vi "LaudaDAQ.vi"(7 "device name":tag="cDAQ9188XT-1C3BF2FMod1") -> (0 "error out":errorcluster, 1 "Tj out":dbl, 2 "data":dynamicdata(waveform), 3 "Sensor OK":bool, 4 "Tj out":dbl, 5 "T external 2":dbl)   [LabVIEW 2016]
panel:
  out "Numeric":dbl
  # "cDAQ9188XT-1C3BF2FMod1"
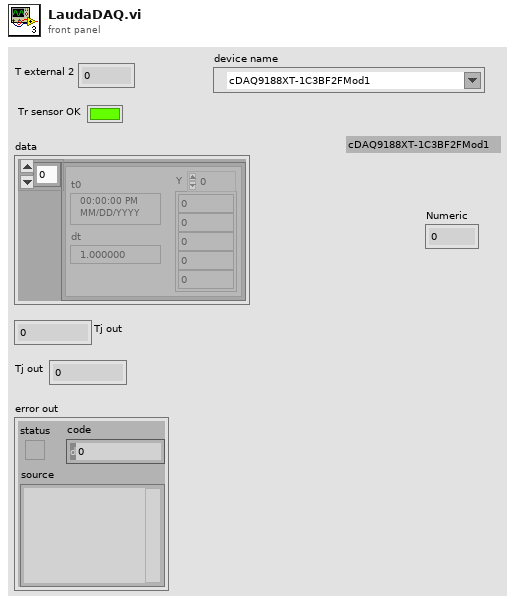
[diagram p1: front panel]
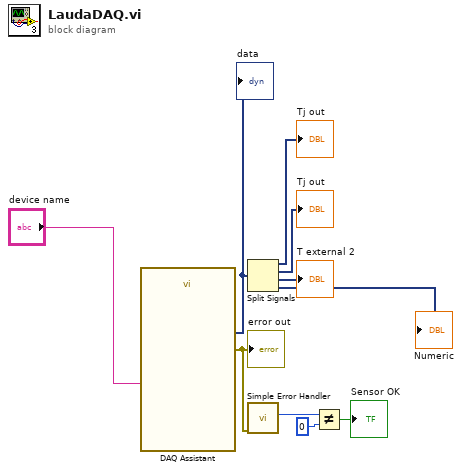
[diagram p0: block diagram]
diagram:
  n1 = call "DAQ Assistant"("device name"="device name") -> ("data"=w10:dynamicdata, "error out"=w3:errorcluster)  [unwired: 16 in, 1 out]
  "error out" <- w3
  "data" <- w10
  n2 = Split Signals(w10) -> (→"Tj out":dynamicdata, →"Tj out":dynamicdata, →"T external 2":dynamicdata, →"Numeric":dynamicdata)  [unwired: 4 in]
  n3 = call <vilib>:"Simple Error Handler.vi"("error in (no error)"=w3) -> ("code out"=w4:i32)  [unwired: 4 in, 4 out]
  n4 = Not Equal?(x=w4, y=0) -> (x != y?=→"Sensor OK":bool)
